vi "Parse Value.vi"(10 "Values":string[](array[string]), 11 "Array":T1[](array[typedef])) -> ()   [LabVIEW 2017]
uses:
  JSON Parsing/Token Types.ctl
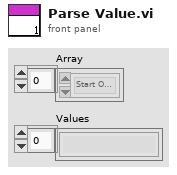
[diagram p1: front panel]
types:
  T1 = typedef "Token Types.ctl" = enum32{"Start Object", "End Object", "Start Array", "End Array", "Colon", "Comma", "Numeric", "true", "false", "null", "String"}
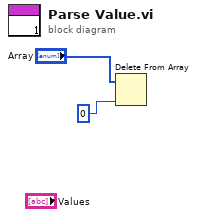
[diagram p0: block diagram]
diagram:
  n1 = Delete From Array(array="Array", index=0 ("length")) -> ()  [unwired: 1 in, 2 out]
